vi "Set TriggerPolarity.vi"(8 "error in (no error)":errorcluster, 10 "TriggerPolarity":i32(ring) items=["ActiveHigh", "ActiveLow"], 11 "TLCamera reference in":refnum<k24>) -> (0 "error out":errorcluster, 3 "TLCamera reference out":refnum<k24>)   [LabVIEW 2015]
uses:
  C:/code/Host/Installer/Scientific Camera Interfaces/LabVIEW/64_bit/Library_X64/Thorlabs.TSI.TLCameraInterfaces.dll
  code/Host/Installer/Scientific Camera Interfaces/LabVIEW/64_bit/Library_X64/Thorlabs.TSI.TLCameraInterfaces.dll
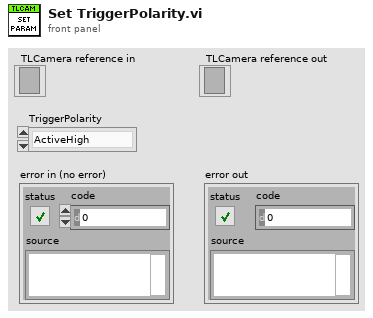
[diagram p1: front panel]
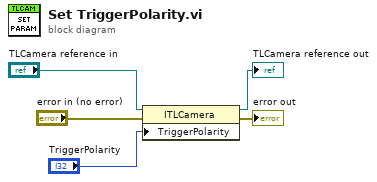
[diagram p0: block diagram]
diagram:
  n1 = property class="ITLCamera"(reference="TLCamera reference in", error in="error in (no error)", "TriggerPolarity"="TriggerPolarity") -> (reference out=→"TLCamera reference out":refnum<k24>, error out=→"error out":errorcluster)
